vi "Database Recordset Properties.vi"(8 "error in (no error)":errorcluster caption="错误输入（无错误）", 11 "Database Recordset 输入":refnum<class "Database Recordset.lvclass"> caption="DNL_LabVIEW Object in") -> (0 "error out":errorcluster caption="错误输出", 1 "recordset properties":T2, 3 "Database Recordset 输出":refnum<class "Database Recordset.lvclass"> caption="DNL_LabVIEW Object out")   [LabVIEW 2011, in "Database Recordset.lvclass"]
uses:
  Database Recordset.lvclass
  <vilib>/addons/database/Auxilliary.llb/DB Tools Cursor Type.ctl
  Database Recordset.lvclass/Database Recordset.ctl
  <vilib>/addons/database/NI_Database_API.lvlib
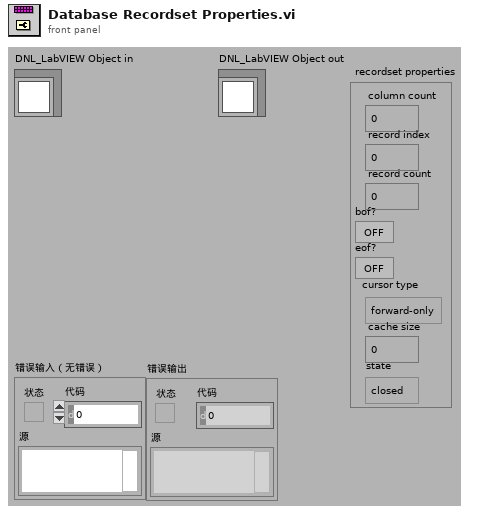
[diagram p1: front panel]
types:
  T1 = typedef "NI_Database_API.lvlib/DB Tools Cursor Type.ctl" = enum16{"forward-only", "keyset", "dynamic", "static"}
  T2 = cluster{"column count":i32, "record index":i32, "record count":i32, "bof?":bool, "eof?":bool, "cursor type":T1, "cache size":i32, "state":enum16{"closed", "open"}}
  T3 = cluster{"Count":i32, "RecordCount":i32, "RecordCount":i32, "BOF":bool, "EOF":bool, "CursorType":i32, "CacheSize":i32, "State":i32}
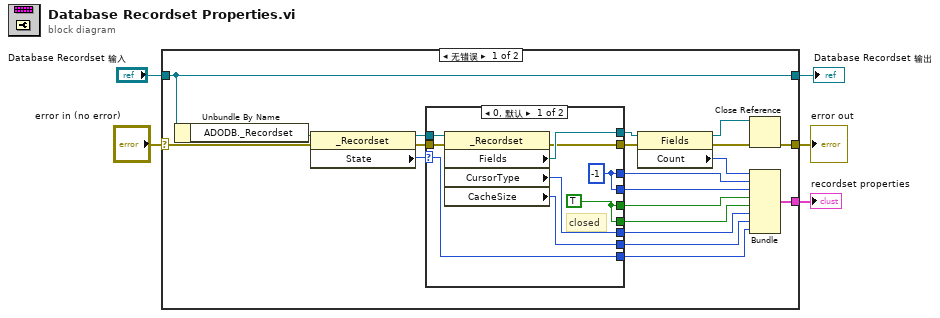
[diagram p0: block diagram]
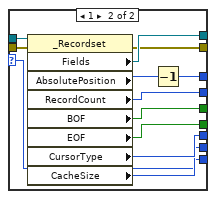
[diagram p2: hidden frame]
diagram:
  n1 = case shown="无错误" "error in (no error)" {
    selector: "error in (no error)" -> [w22 w48]
    tunnel: [w13 w48] -> w4
    tunnel: [w19 w47] -> w2
    tunnel: "Database Recordset 输入" -> [w19 w47]
    tunnel: [w25 _] -> w1
    frame No Error {
      n2 = Unbundle By Name(w19) -> ("ADODB._Recordset"=w24:refnum<k7>)
      n3 = property class="_Recordset"(reference=w24, error in=w22) -> (reference out=w21:refnum<k7>, error out=w20:errorcluster, "State"=w23:i32)
      n4 = case shown="0, 默认" w23 {
        selector: w23 -> [w32 w40]
        tunnel: [w34 w46] -> w17
        tunnel: [w33 w45] -> w16
        tunnel: [w28 w39] -> w11
        tunnel: [w29 w44] -> w10
        tunnel: [w29 w43] -> w9
        tunnel: [w30 w42] -> w8
        tunnel: [w31 w41] -> w7
        tunnel: [w32 w40] -> w6
        tunnel: [w28 w37] -> w12
        tunnel: w21 -> [w27 w36]
        tunnel: w20 -> [w26 w35]
        frame 0, Default {
          w28 = -1 ("RecordCount")
          w29 = TRUE ("EOF")
          # "closed"
          n5 = property class="_Recordset"(reference=w27, error in=w26) -> (error out=w33:errorcluster, "Fields"=w34:refnum<k7>, "CursorType"=w30:i32, "CacheSize"=w31:i32)  [unwired: 1 out]
        }
        frame 1 {
          n6 = property class="_Recordset"(reference=w36, error in=w35) -> (error out=w45:errorcluster, "Fields"=w46:refnum<k7>, "AbsolutePosition"=w38:i32, "RecordCount"=w39:i32, "BOF"=w44:bool, "EOF"=w43:bool, "CursorType"=w42:i32, "CacheSize"=w41:i32)  [unwired: 1 out]
          n7 = Decrement(x=w38) -> (x-1=w37:i32)
        }
      }
      n8 = property class="Fields"(reference=w17, error in=w16) -> (reference out=w15:refnum<k7>, error out=w14:errorcluster, "Count"=w18:i32)
      n9 = Close Reference(reference=w15, error in (no error)=w14) -> (error out=w13:errorcluster)
      n10 = Bundle("Count"=w18, "RecordCount"=w12, "RecordCount"=w11, "BOF"=w10, "EOF"=w9, "CursorType"=w8, "CacheSize"=w7, "State"=w6) -> (w25:T3)  [unwired: 1 out]
    }
    frame Error {
    }
  }
  "error out" <- w4
  "Database Recordset 输出" <- w2
  "recordset properties" <- w1
